vi "Initiailize_Statistical_Values_2.vi"() -> (0 "Statistics":T1)   [LabVIEW 2013]
panel:
  in  "Mean Path Velo\ncities for Tracks":dbl[](array[numeric])
  in  "Track length in pixels":dbl[](array[numeric])
  in  "Track duration in frames":u16[](array[numeric])
  in  "Mean Instant Velo\ncities for Tracks":dbl[](array[numeric])
  in  "Tracks in columns":dbl[][](array[numeric])
  in  "Path Velocities (All)":dbl[](array[numeric])
  in  "Instant Velocities (All)":dbl[](array[numeric])
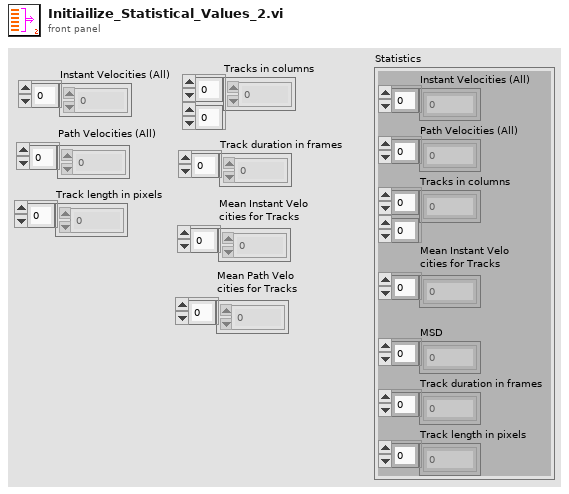
[diagram p1: front panel]
types:
  T1 = cluster{"Instant Velocities (All)":dbl[], "Path Velocities (All) ":dbl[], "Tracks in columns":dbl[][], "Mean Instant Velo\ncities for Tracks":dbl[], "MSD":dbl[], "Track duration in frames":u16[], "Track length in pixels":dbl[]}
  T2 = cluster{"Instant Velocities (All)":dbl[], "Path Velocities (All) ":dbl[], "Tracks in columns":dbl[][], "Mean Instant Velo\ncities for Tracks":dbl[], "Mean Path Velo\ncities for Tracks":dbl[], "Track duration in frames":u16[], "Track length in pixels":dbl[]}
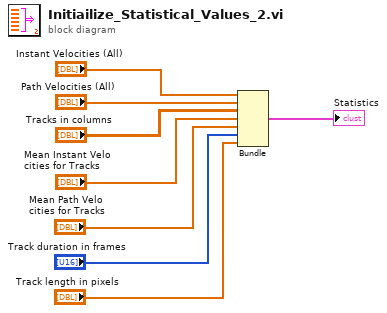
[diagram p0: block diagram]
diagram:
  n1 = Bundle("Instant Velocities (All)"="Instant Velocities (All)", "Path Velocities (All)"="Path Velocities (All)", "Tracks in columns"="Tracks in columns", "Mean Instant Velo\ncities for Tracks"="Mean Instant Velo\ncities for Tracks", "Mean Path Velo\ncities for Tracks"="Mean Path Velo\ncities for Tracks", "Track duration in frames"="Track duration in frames", "Track length in pixels"="Track length in pixels") -> (→"Statistics":T2)  [unwired: 1 in]
